vi "QuickChangeParameters Example.vi"() -> ()   [LabVIEW 2015]
uses:
  <userlib>/836 Library/System/QCP Support Code/QCP_Get_I32.vi
  <userlib>/836 Library/System/QCP Support Code/QCP_Get_DBL.vi
  <userlib>/836 Library/System/QCP Support Code/QCP_Get_STR.vi
  <userlib>/836 Library/System/QCP Support Code/QCP_Set_I32.vi
  <userlib>/836 Library/System/QCP Support Code/QCP_Set_DBL.vi
  <userlib>/836 Library/System/QCP Support Code/QCP_Set_STR.vi
panel:
  in  "Eleanor":string="Soccer"
  in  "Jeanette":dbl=3.141592653589793
  in  "Brittany":i32=2
  out "Theodore":string
  out "Simon":dbl=inf
  in  "Read File":bool
  in  "Write File":bool
  out "Alvin":i32=2147483647
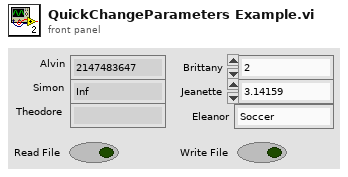
[diagram p1: front panel]
types:
  T1 = typedef "QCP Data Block.ctl" = refnum<data-value>
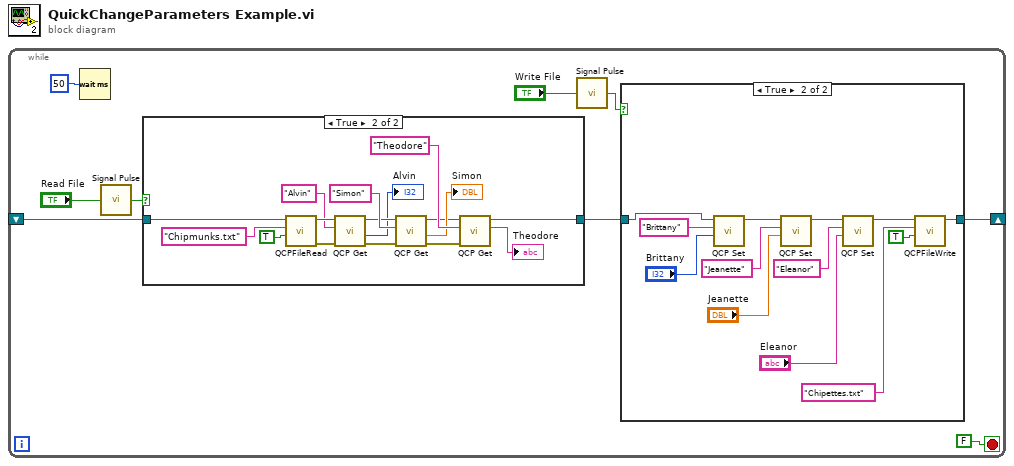
[diagram p0: block diagram]
diagram:
  n1 = while {
    shift-right: [w6] -> _
    shift-left: _ -> [w7]
    stop <- FALSE stop-if-true
    n2 = Wait (ms)(milliseconds to wait=u32 50) -> ()  [unwired: 1 out]
    n3 = call <userlib>:"Signal Pulse.vi"("Input"="Read File") -> ("Output"=w3:bool)
    n4 = case shown="True" w3 {
      tunnel: w7 -> [w24 w40]
      tunnel: [w24 w27] -> w5
      frame False {
      }
      frame True {
        n5 = call <userlib>:"QCPFileRead.vi"("Path Relative?"=TRUE, "File Path"="Chipmunks.txt", "QCP Data Block In"=w40) -> ("error out"=w26:errorcluster, "QCP Data Block Out"=w34:T1)  [unwired: 7 in]
        n6 = call-poly <userlib>:"QCP Get.vi"("QCP Data Block In"=w34, "QCP Name"="Alvin", "Error In"=w26) -> ("QCP Data Block Out"=w33:T1, "Value Out"=→"Alvin":i32, "Error Out"=w30:errorcluster)  [unwired: 5 in]
        n7 = call-poly <userlib>:"QCP Get.vi"("QCP Data Block In"=w33, "QCP Name"="Simon", "Error In"=w30) -> ("QCP Data Block Out"=w28:T1, "Value Out"=→"Simon":dbl, "Error Out"=w29:errorcluster)  [unwired: 5 in]
        n8 = call-poly <userlib>:"QCP Get.vi"("QCP Data Block In"=w28, "QCP Name"="Theodore", "Error In"=w29) -> ("QCP Data Block Out"=w27:T1, "Value Out"=→"Theodore":string)  [unwired: 5 in, 1 out]
      }
    }
    n9 = call <userlib>:"Signal Pulse.vi"("Input"="Write File") -> ("Output"=w1:bool)
    n10 = case shown="True" w1 {
      tunnel: [w10 w23] -> w6
      tunnel: w5 -> [w10 w11]
      frame False {
      }
      frame True {
        n11 = call-poly <userlib>:"QCP Set.vi"("QCP Data Block In"=w11, "QCP Name"="Brittany", "Value In"="Brittany") -> ("QCP Data Block Out"=w18:T1)  [unwired: 7 in]
        n12 = call-poly <userlib>:"QCP Set.vi"("QCP Data Block In"=w18, "QCP Name"="Jeanette", "Value In"="Jeanette") -> ("QCP Data Block Out"=w16:T1)  [unwired: 7 in]
        n13 = call-poly <userlib>:"QCP Set.vi"("QCP Data Block In"=w16, "QCP Name"="Eleanor", "Value In"="Eleanor") -> ("QCP Data Block Out"=w14:T1)  [unwired: 7 in]
        n14 = call <userlib>:"QCPFileWrite.vi"("Path Relative?"=TRUE, "File Path"="Chipettes.txt", "QCP Data Block In"=w14) -> ("QCP Data Block Out"=w23:T1)  [unwired: 7 in, 1 out]
      }
    }
  }
